vi "Stop_Synthesis.vi"(0 "TCP connection ID":refnum<k5>, 12 "error in":errorcluster) -> (4 "TCP connection ID out":refnum<k5>, 14 "error out":errorcluster)   [LabVIEW 2017]
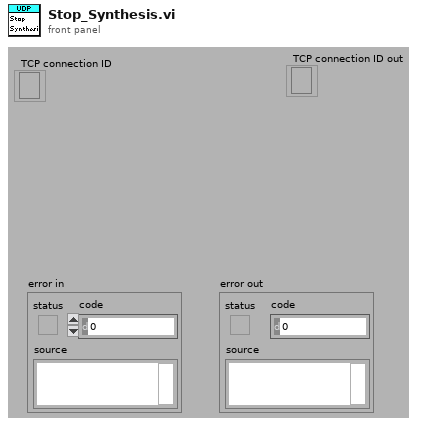
[diagram p1: front panel]
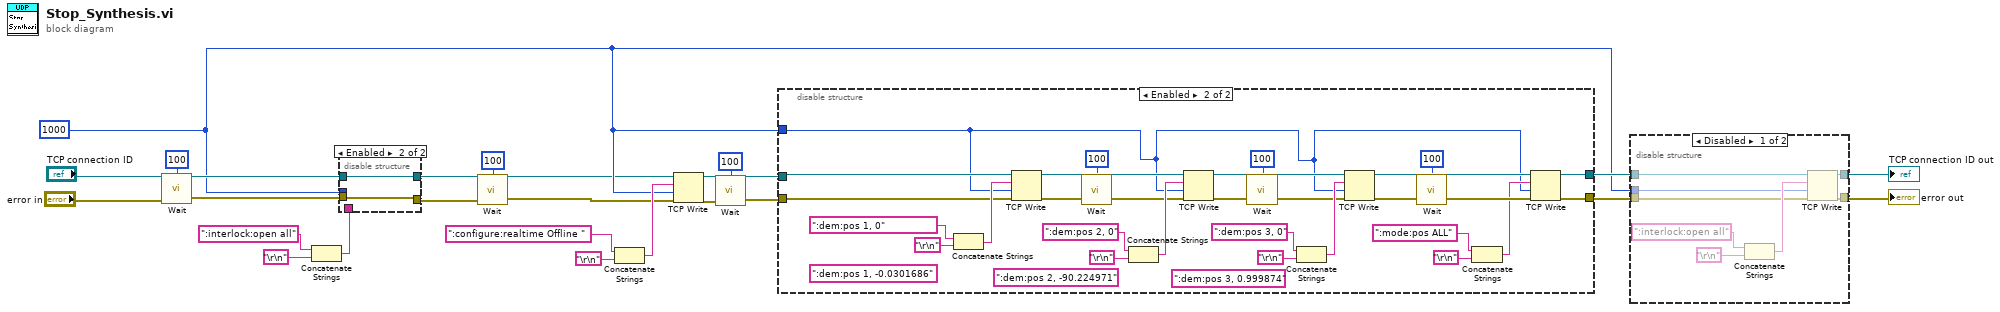
[diagram p0: block diagram]
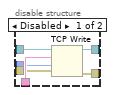
[diagram p2: hidden frame]
diagram:
  w8 = 1000 ("Acutrol NodeID")
  n1 = call "Wait.vi"("Wartezeit in ms"=u32 100, "error in (no error)"="error in") -> ("error out"=w1:errorcluster)  [unwired: 3 in]
  n2 = Concatenate Strings(":interlock:open all" ("ACL Command"), "\r\n") -> (w10:string)
  n3 = disable-structure shown="Enabled" {
    disable-tunnel: w10 -> [w29 _]
    disable-tunnel: "TCP connection ID" -> [w28 w31]
    disable-tunnel: w8 -> [w27 _]
    disable-tunnel: [w26 w31] -> w6
    disable-tunnel: [w25 w30] -> w5
    disable-tunnel: w1 -> [w24 w30]
    frame Disabled {
      n4 = TCP Write(connection ID=w28, data in=w29, error in (no error)=w24, 9:w27) -> (connection ID out=w26:refnum<k5>, error out=w25:errorcluster)  [unwired: 1 out]
    }
    frame Enabled {
    }
  }
  n5 = call "Wait.vi"("Wartezeit in ms"=u32 100, "error in (no error)"=w5) -> ("error out"=w4:errorcluster)  [unwired: 3 in]
  n6 = Concatenate Strings(":configure:realtime Offline " ("ACL Command"), "\r\n") -> (w17:string)
  n7 = TCP Write(connection ID=w6, data in=w17, error in (no error)=w4, 9:w8) -> (connection ID out=w16:refnum<k5>, error out=w21:errorcluster)  [unwired: 1 out]
  n8 = call "Wait.vi"("Wartezeit in ms"=u32 100, "error in (no error)"=w21) -> ("error out"=w15:errorcluster)  [unwired: 3 in]
  n9 = disable-structure shown="Enabled" {
    disable-tunnel: [w33 w34] -> w23
    disable-tunnel: [w32 w35] -> w22
    disable-tunnel: w16 -> [w32 w38]
    disable-tunnel: w8 -> [_ w36]
    disable-tunnel: w15 -> [w33 w37]
    frame Disabled {
    }
    frame Enabled {
      (unwired) ":dem:pos 3, 0.999874" ("ACL Command")
      (unwired) ":dem:pos 2, -90.224971" ("ACL Command")
      (unwired) ":dem:pos 1, -0.0301686" ("ACL Command")
      n10 = Concatenate Strings(":dem:pos 1, 0" ("ACL Command"), "\r\n") -> (w57:string)
      n11 = TCP Write(connection ID=w38, data in=w57, error in (no error)=w37, 9:w36) -> (connection ID out=w58:refnum<k5>, error out=w41:errorcluster)  [unwired: 1 out]
      n12 = call "Wait.vi"("Wartezeit in ms"=u32 100, "error in (no error)"=w41) -> ("error out"=w39:errorcluster)  [unwired: 3 in]
      n13 = Concatenate Strings(":dem:pos 2, 0" ("ACL Command"), "\r\n") -> (w56:string)
      n14 = TCP Write(connection ID=w58, data in=w56, error in (no error)=w39, 9:w36) -> (connection ID out=w59:refnum<k5>, error out=w44:errorcluster)  [unwired: 1 out]
      n15 = call "Wait.vi"("Wartezeit in ms"=u32 100, "error in (no error)"=w44) -> ("error out"=w43:errorcluster)  [unwired: 3 in]
      n16 = Concatenate Strings(":dem:pos 3, 0" ("ACL Command"), "\r\n") -> (w55:string)
      n17 = TCP Write(connection ID=w59, data in=w55, error in (no error)=w43, 9:w36) -> (connection ID out=w62:refnum<k5>, error out=w46:errorcluster)  [unwired: 1 out]
      n18 = call "Wait.vi"("Wartezeit in ms"=u32 100, "error in (no error)"=w46) -> ("error out"=w61:errorcluster)  [unwired: 3 in]
      n19 = Concatenate Strings(":mode:pos ALL" ("ACL Command"), "\r\n") -> (w54:string)
      n20 = TCP Write(connection ID=w62, data in=w54, error in (no error)=w61, 9:w36) -> (connection ID out=w35:refnum<k5>, error out=w34:errorcluster)  [unwired: 1 out]
    }
  }
  n21 = disable-structure shown="Disabled" {
    disable-tunnel: w23 -> [w67 w71]
    disable-tunnel: w22 -> [w66 w72]
    disable-tunnel: w8 -> [w65 _]
    disable-tunnel: [w64 w72] -> w14
    disable-tunnel: [w63 w71] -> w13
    frame Disabled {
      n22 = Concatenate Strings(":interlock:open all" ("ACL Command"), "\r\n") -> (w68:string)
      n23 = TCP Write(connection ID=w66, data in=w68, error in (no error)=w67, 9:w65) -> (connection ID out=w64:refnum<k5>, error out=w63:errorcluster)  [unwired: 1 out]
    }
    frame Enabled {
    }
  }
  "error out" <- w13
  "TCP connection ID out" <- w14
